vi "Is IPv4 address.vi"(8 "error in (no error)":errorcluster, 11 "address string":string) -> (0 "error out":errorcluster, 3 "address U32":u32)   [LabVIEW 2020, in "NI_WFCN.lvlib"]
doc: "Attempts to parse the specified string as an IPv4 dotted quad, or returns error on failure.\n\nThe difference between this VI and the String To IP primitive is that this VI is guaranteed to not attempt a DNS lookup."
uses:
  <vilib>/net/WFCN/NI_WFCN.lvlib
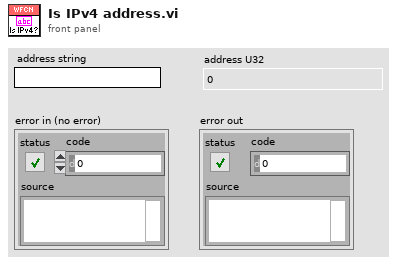
[diagram p1: front panel]
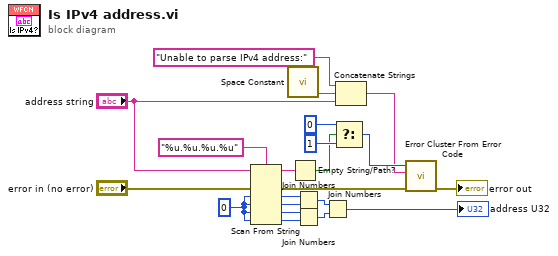
[diagram p0: block diagram]
diagram:
  w13 = u8 0
  n1 = Scan From String(format string="%u.%u.%u.%u", input string="address string", error in="error in (no error)", default 1=w13, default 2=w13, default 3=w13, default 4=w13) -> (remaining string=w15:string, error out=w20:errorcluster, output 1=w12:u8, output 2=w11:u8, output 3=w10:u8, output 4=w9:u8)  [unwired: 1 in, 1 out]
  n2 = call <vilib>:"Space Constant.vi"() -> ("String"=w2:string)
  n3 = Empty String/Path?(string/path=w15) -> (empty?=w17:bool)
  n4 = Join Numbers(hi=w12, lo=w11) -> ((hi.lo)=w8:u16)
  n5 = Join Numbers(hi=w10, lo=w9) -> ((hi.lo)=w7:u16)
  n6 = Join Numbers(hi=w8, lo=w7) -> ((hi.lo)=→"address U32":u32)
  n7 = Select(t=0, s=w17, f=1) -> (s? t:f=w21:i32)
  n8 = Concatenate Strings("Unable to parse IPv4 address:" ("string"), w2, "address string") -> (w3:string)
  n9 = call <vilib>:"Error Cluster From Error Code.vi"("error in (no error)"=w20, "error message (\"\")"=w3, "error code (0)"=w21) -> ("error out"=→"error out":errorcluster)  [unwired: 6 in]
